vi "Agilent 34970 Adjust Gain.vi"(8 "Error In":errorcluster, 11 "Input Channel":string="(5) 107 ") -> (0 "Error Out":errorcluster, 1 "Output Channel":string="107", 2 "Offset":dbl, 3 "Output Gain":dbl=5.0, 5 "Name":string)   [LabVIEW 2016]
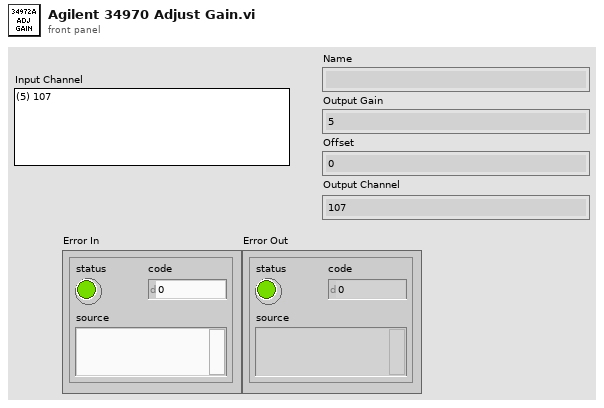
[diagram p1: front panel]
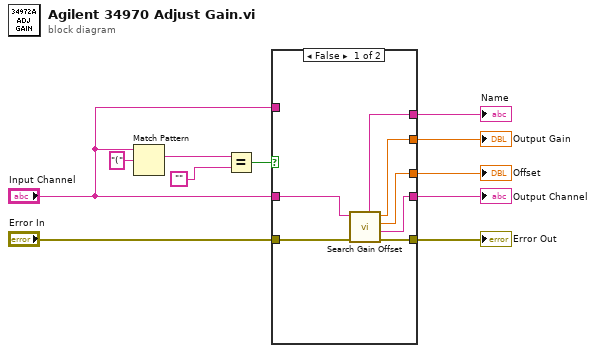
[diagram p0: block diagram]
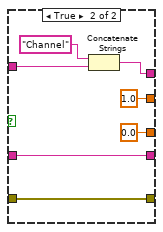
[diagram p2: hidden frame]
diagram:
  n1 = Match Pattern(string="Input Channel", regular expression="(") -> (match substring=w5:string)  [unwired: 1 in, 3 out]
  n2 = Equal?(x=w5, y="") -> (x = y?=w3:bool)
  n3 = case shown="False" w3 {
    tunnel: "Error In" -> [w18 w23]
    tunnel: [w17 w23] -> w10
    tunnel: [w16 w25] -> w9
    tunnel: [w15 1.0 ("Gain")] -> w8
    tunnel: [w14 0.0 ("Offset")] -> w7
    tunnel: "Input Channel" -> [w13 w25]
    tunnel: [w12 w19] -> w2
    tunnel: "Input Channel" -> [_ w20]
    frame False {
      n4 = call "Search Gain Offset.vi"("Error In"=w18, "Input Channel"=w13) -> ("Error Out"=w17:errorcluster, "Channel"=w16:string, "Offset"=w14:dbl, "Gain"=w15:dbl, "Name"=w12:string)  [unwired: 5 in]
    }
    frame True {
      n5 = Concatenate Strings("Channel" ("string"), w20) -> (w19:string)
    }
  }
  "Output Gain" <- w8
  "Output Channel" <- w9
  "Error Out" <- w10
  "Offset" <- w7
  "Name" <- w2
